vi "_RT Global.vi"() -> ()   [LabVIEW 2018]
uses:
  Type/_RT Instrument 2.ctl
  Type/_RT Configuration 2.ctl
  Type/_RT Startup Options.ctl
  Type/_RT Instrument State.ctl
  Type/FPGA Typedef.ctl
panel:
  out "Leybold Pump ON":bool
  out "Tuning Error Generated":bool
  out "Exhaust gas error":bool
  out "ScanParam":bool
  out "UseLeybold":bool
  out "FPGA Ref":T1
  out "IgnoreError":bool
  out "Simulation":bool
  out "Single Source":bool
  out "FPGA semaphore":T2
  out "Ele On":bool
  out "semaphore":T2
  out "RT Time(s)":dbl=432.2503070831299
  out "ADC Values":i32[](array[numeric])=[0, 0, 0, 0, 0, 0, 0, 0, 0, 0, 0, 0, 0, 0, 0, 0, 0, 0, 0, 0, 0, 0, 0, 0, 0, 0, 0, 0, 0, 0, 0, 0, 0, 0, 0, 0, 0, 0, 0, 0, 0, 0, 0, 0, 0, 0, 0, 0, 0, 0, 0, 0, 0, 0, 0, 0, 0, 0, 0, 0, 0, 0, 0, 0, 0, 0, 0, 0, 0, 0, 0, 0, 0, 0, 0, 0, 0, 0, 0, 0, 0, 0, 0, 0, 0, 0, 0, 0, 0, 0, 0, 0, 0, 0, 0, 0, 0, 0, 0, 0, 0, 0, 0, 0, 0, 0, 0, 0, 0, 0, 0, 0, 0, 0, 0, 0, 0, 0, 0, 0, 0, 0, 1, 0, 1, 0, 0, 0]
  out "StartupMode":u8=2
  out "InstrState":T3=enum."Mass Spectrometer is Off"
  in  "ADC Table":T4[](array[typedef])=[{"Name"="DET HORN, 6KV", "Ch#"=0, "Min"=0.0, "Max"=0.0, "Def+"=0.0, "Def-"=0.0, "Offset"=0.0, "Slope"=33.0, "Type"=0, "Description"="", "SettleT"=0.0}, {"Name"="DET BIAS, KV", "Ch#"=0, "Min"=0.0, "Max"=0.0, "Def+"=0.0, "Def-"=0.0, "Offset"=0.0, "Slope"=33.0, "Type"=0, "Description"="", "SettleT"=0.0}, {"Name"="Discriminator", "Ch#"=0, "Min"=0.0, "Max"=0.0, "Def+"=0.0, "Def-"=0.0, "Offset"=4.0, "Slope"=1100.0, "Type"=0, "Description"="", "SettleT"=0.0}, {"Name"="DET Spare4", "Ch#"=0, "Min"=0.0, "Max"=0.0, "Def+"=0.0, "Def-"=0.0, "Offset"=0.0, "Slope"=1.0, "Type"=0, "Description"="", "SettleT"=0.0}, {"Name"="DET Spare5", "Ch#"=0, "Min"=0.0, "Max"=0.0, "Def+"=0.0, "Def-"=0.0, "Offset"=0.0, "Slope"=1.0, "Type"=0, "Description"="", "SettleT"=0.0}, {"Name"="DET Spare6", "Ch#"=0, "Min"=0.0, "Max"=0.0, "Def+"=0.0, "Def-"=0.0, "Offset"=0.0, "Slope"=1.0, "Type"=0, "Description"="", "SettleT"=0.0}, {"Name"="DET Spare7", "Ch#"=0, "Min"=0.0, "Max"=0.0, "Def+"=0.0, "Def-"=0.0, "Offset"=0.0, "Slope"=1.0, "Type"=0, "Description"="", "SettleT"=0.0}, {"Name"="DET Spare8", "Ch#"=0, "Min"=0.0, "Max"=0.0, "Def+"=0.0, "Def-"=0.0, "Offset"=0.0, "Slope"=1.0, "Type"=0, "Description"="", "SettleT"=0.0}, {"Name"="LV PS CUR, 10A", "Ch#"=0, "Min"=0.0, "Max"=0.0, "Def+"=0.0, "Def-"=0.0, "Offset"=0.0, "Slope"=1.0, "Type"=0, "Description"="", "SettleT"=0.0}, {"Name"="RPUMP CUR, 30A", "Ch#"=0, "Min"=0.0, "Max"=0.0, "Def+"=0.0, "Def-"=0.0, "Offset"=0.0, "Slope"=1.0, "Type"=0, "Description"="", "SettleT"=0.0}, {"Name"="AC box Spare3", "Ch#"=0, "Min"=0.0, "Max"=0.0, "Def+"=0.0, "Def-"=0.0, "Offset"=0.0, "Slope"=1.0, "Type"=0, "Description"="", "SettleT"=0.0}, {"Name"="AC box Spare4", "Ch#"=0, "Min"=0.0, "Max"=0.0, "Def+"=0.0, "Def-"=0.0, "Offset"=0.0, "Slope"=1.0, "Type"=0, "Description"="", "SettleT"=0.0}, {"Name"="AC box Spare5", "Ch#"=0, "Min"=0.0, "Max"=0.0, "Def+"=0.0, "Def-"=0.0, "Offset"=0.0, "Slope"=1.0, "Type"=0, "Description"="", "SettleT"=0.0}, {"Name"="AC box Spare6", "Ch#"=0, "Min"=0.0, "Max"=0.0, "Def+"=0.0, "Def-"=0.0, "Offset"=0.0, "Slope"=1.0, "Type"=0, "Description"="", "SettleT"=0.0}, {"Name"="HTR PS CUR, 10A", "Ch#"=0, "Min"=0.0, "Max"=0.0, "Def+"=0.0, "Def-"=0.0, "Offset"=0.0, "Slope"=1.0, "Type"=0, "Description"="", "SettleT"=0.0}, {"Name"="TRB PS CUR, 5A", "Ch#"=0, "Min"=0.0, "Max"=0.0, "Def+"=0.0, "Def-"=0.0, "Offset"=0.0, "Slope"=1.0, "Type"=0, "Description"="", "SettleT"=0.0}, {"Name"="Q1 DC POLE A, V", "Ch#"=0, "Min"=0.0, "Max"=0.0, "Def+"=0.0, "Def-"=0.0, "Offset"=0.5, "Slope"=402.0, "Type"=0, "Description"="", "SettleT"=0.0}, {"Name"="Q1 DC POLE B, V", "Ch#"=0, "Min"=0.0, "Max"=0.0, "Def+"=0.0, "Def-"=0.0, "Offset"=0.5, "Slope"=402.0, "Type"=0, "Description"="", "SettleT"=0.0}, {"Name"="Q2 DC POLE A, V", "Ch#"=0, "Min"=0.0, "Max"=0.0, "Def+"=0.0, "Def-"=0.0, "Offset"=0.5, "Slope"=402.0, "Type"=0, "Description"="", "SettleT"=0.0}, {"Name"="Q2 DC POLE B, V", "Ch#"=0, "Min"=0.0, "Max"=0.0, "Def+"=0.0, "Def-"=0.0, "Offset"=0.5, "Slope"=402.0, "Type"=0, "Description"="", "SettleT"=0.0}, {"Name"="DC Spare5", "Ch#"=0, "Min"=0.0, "Max"=0.0, "Def+"=0.0, "Def-"=0.0, "Offset"=0.0, "Slope"=1.0, "Type"=0, "Description"="", "SettleT"=0.0}, {"Name"="DC Spare6", "Ch#"=0, "Min"=0.0, "Max"=0.0, "Def+"=0.0, "Def-"=0.0, "Offset"=0.0, "Slope"=1.0, "Type"=0, "Description"="", "SettleT"=0.0}, {"Name"="DC Spare7", "Ch#"=0, "Min"=0.0, "Max"=0.0, "Def+"=0.0, "Def-"=0.0, "Offset"=0.0, "Slope"=1.0, "Type"=0, "Description"="", "SettleT"=0.0}, {"Name"="DC Spare8", "Ch#"=0, "Min"=0.0, "Max"=0.0, "Def+"=0.0, "Def-"=0.0, "Offset"=0.0, "Slope"=1.0, "Type"=0, "Description"="", "SettleT"=0.0}, {"Name"="Q2 RF Pk-Pk, V", "Ch#"=0, "Min"=0.0, "Max"=0.0, "Def+"=0.0, "Def-"=0.0, "Offset"=0.0, "Slope"=-1208.0, "Type"=0, "Description"="", "SettleT"=0.0}, {"Name"="Q2 RF HS1 TEMP, C", "Ch#"=0, "Min"=0.0, "Max"=90.0, "Def+"=0.0, "Def-"=0.0, "Offset"=0.0, "Slope"=100.0, "Type"=0, "Description"="", "SettleT"=0.0}, {"Name"="Q2 RF HS2 TEMP, C", "Ch#"=0, "Min"=0.0, "Max"=0.0, "Def+"=0.0, "Def-"=0.0, "Offset"=0.0, "Slope"=100.0, "Type"=0, "Description"="", "SettleT"=0.0}, {"Name"="Q2 TUNING DC, V", "Ch#"=0, "Min"=0.0, "Max"=0.0, "Def+"=0.0, "Def-"=0.0, "Offset"=0.0, "Slope"=3.0, "Type"=0, "Description"="", "SettleT"=0.0}, {"Name"="Q2 RF Spare5", "Ch#"=0, "Min"=0.0, "Max"=0.0, "Def+"=0.0, "Def-"=0.0, "Offset"=0.0, "Slope"=1.0, "Type"=0, "Description"="", "SettleT"=0.0}, {"Name"="Q2 RF Spare6", "Ch#"=0, "Min"=0.0, "Max"=0.0, "Def+"=0.0, "Def-"=0.0, "Offset"=0.0, "Slope"=1.0, "Type"=0, "Description"="", "SettleT"=0.0}, {"Name"="Q2 RF Spare7", "Ch#"=0, "Min"=0.0, "Max"=0.0, "Def+"=0.0, "Def-"=0.0, "Offset"=0.0, "Slope"=1.0, "Type"=0, "Description"="", "SettleT"=0.0}, {"Name"="Q2 RF Spare8", "Ch#"=0, "Min"=0.0, "Max"=0.0, "Def+"=0.0, "Def-"=0.0, "Offset"=0.0, "Slope"=1.0, "Type"=0, "Description"="", "SettleT"=0.0}, {"Name"="CC AF +/-400, V", "Ch#"=0, "Min"=0.0, "Max"=0.0, "Def+"=0.0, "Def-"=0.0, "Offset"=1.0, "Slope"=402.0, "Type"=0, "Description"="", "SettleT"=0.0}, {"Name"="L2 +/-400, V", "Ch#"=0, "Min"=0.0, "Max"=0.0, "Def+"=0.0, "Def-"=0.0, "Offset"=1.0, "Slope"=402.0, "Type"=0, "Description"="", "SettleT"=0.0}, {"Name"="PF +/-400, V", "Ch#"=0, "Min"=0.0, "Max"=0.0, "Def+"=0.0, "Def-"=0.0, "Offset"=1.0, "Slope"=402.0, "Type"=0, "Description"="", "SettleT"=0.0}, {"Name"="CC L1 +/-400, V", "Ch#"=0, "Min"=0.0, "Max"=0.0, "Def+"=0.0, "Def-"=0.0, "Offset"=1.0, "Slope"=402.0, "Type"=0, "Description"="", "SettleT"=0.0}, {"Name"="CC L2 +/-400, V", "Ch#"=0, "Min"=0.0, "Max"=0.0, "Def+"=0.0, "Def-"=0.0, "Offset"=1.0, "Slope"=402.0, "Type"=0, "Description"="", "SettleT"=0.0}, {"Name"="CC L3 +/-400, V", "Ch#"=0, "Min"=0.0, "Max"=0.0, "Def+"=0.0, "Def-"=0.0, "Offset"=1.0, "Slope"=404.0, "Type"=0, "Description"="", "SettleT"=0.0}, {"Name"="CC L4 +/-400, V", "Ch#"=0, "Min"=0.0, "Max"=0.0, "Def+"=0.0, "Def-"=0.0, "Offset"=1.0, "Slope"=404.0, "Type"=0, "Description"="", "SettleT"=0.0}, {"Name"="ID +/-400, V", "Ch#"=0, "Min"=0.0, "Max"=0.0, "Def+"=0.0, "Def-"=0.0, "Offset"=1.0, "Slope"=404.0, "Type"=0, "Description"="", "SettleT"=0.0}, {"Name"="L1 +/-400, V", "Ch#"=0, "Min"=0.0, "Max"=0.0, "Def+"=0.0, "Def-"=0.0, "Offset"=1.0, "Slope"=400.0, "Type"=0, "Description"="", "SettleT"=0.0}, {"Name"="M1 +/-400, V", "Ch#"=0, "Min"=0.0, "Max"=0.0, "Def+"=0.0, "Def-"=0.0, "Offset"=1.0, "Slope"=402.0, "Type"=0, "Description"="", "SettleT"=0.0}, {"Name"="EV +/-400, V", "Ch#"=0, "Min"=0.0, "Max"=0.0, "Def+"=0.0, "Def-"=0.0, "Offset"=4.0, "Slope"=404.0, "Type"=0, "Description"="", "SettleT"=0.0}, {"Name"="Spare +/-400, V", "Ch#"=0, "Min"=0.0, "Max"=0.0, "Def+"=0.0, "Def-"=0.0, "Offset"=1.0, "Slope"=402.0, "Type"=0, "Description"="", "SettleT"=0.0}, {"Name"="M2 +/-400, V", "Ch#"=0, "Min"=0.0, "Max"=0.0, "Def+"=0.0, "Def-"=0.0, "Offset"=3.0, "Slope"=404.0, "Type"=0, "Description"="", "SettleT"=0.0}, {"Name"="CC +/-400, V", "Ch#"=0, "Min"=0.0, "Max"=0.0, "Def+"=0.0, "Def-"=0.0, "Offset"=1.0, "Slope"=404.0, "Type"=0, "Description"="", "SettleT"=0.0}, {"Name"="Spare +/-400, V", "Ch#"=0, "Min"=0.0, "Max"=0.0, "Def+"=0.0, "Def-"=0.0, "Offset"=0.0, "Slope"=404.0, "Type"=0, "Description"="", "SettleT"=0.0}, {"Name"="Spare +/-400, V", "Ch#"=0, "Min"=0.0, "Max"=0.0, "Def+"=0.0, "Def-"=0.0, "Offset"=-1.5, "Slope"=404.0, "Type"=0, "Description"="", "SettleT"=0.0}, {"Name"="Q1 RF Pk-Pk, V", "Ch#"=0, "Min"=0.0, "Max"=0.0, "Def+"=0.0, "Def-"=0.0, "Offset"=0.0, "Slope"=-1221.0, "Type"=0, "Description"="", "SettleT"=0.0}, {"Name"="Q1 RF HS1 TEMP, C", "Ch#"=0, "Min"=0.0, "Max"=0.0, "Def+"=0.0, "Def-"=0.0, "Offset"=0.0, "Slope"=100.0, "Type"=0, "Description"="", "SettleT"=0.0}, {"Name"="Q1 RF HS2 TEMP, C", "Ch#"=0, "Min"=0.0, "Max"=0.0, "Def+"=0.0, "Def-"=0.0, "Offset"=0.0, "Slope"=100.0, "Type"=0, "Description"="", "SettleT"=0.0}, {"Name"="Q1 TUNING DC, V", "Ch#"=0, "Min"=0.0, "Max"=0.0, "Def+"=0.0, "Def-"=0.0, "Offset"=0.0, "Slope"=3.0, "Type"=0, "Description"="", "SettleT"=0.0}, {"Name"="Q1 RF Spare5", "Ch#"=0, "Min"=0.0, "Max"=0.0, "Def+"=0.0, "Def-"=0.0, "Offset"=0.0, "Slope"=1.0, "Type"=0, "Description"="", "SettleT"=0.0}, {"Name"="Q1 RF Spare6", "Ch#"=0, "Min"=0.0, "Max"=0.0, "Def+"=0.0, "Def-"=0.0, "Offset"=0.0, "Slope"=1.0, "Type"=0, "Description"="", "SettleT"=0.0}, {"Name"="Q1 RF Spare7", "Ch#"=0, "Min"=0.0, "Max"=0.0, "Def+"=0.0, "Def-"=0.0, "Offset"=0.0, "Slope"=1.0, "Type"=0, "Description"="", "SettleT"=0.0}, {"Name"="Q1 RF Spare8", "Ch#"=0, "Min"=0.0, "Max"=0.0, "Def+"=0.0, "Def-"=0.0, "Offset"=0.0, "Slope"=1.0, "Type"=0, "Description"="", "SettleT"=0.0}, {"Name"="M1 RF Pk-Pk, V", "Ch#"=0, "Min"=0.0, "Max"=0.0, "Def+"=0.0, "Def-"=0.0, "Offset"=0.0, "Slope"=-885.0, "Type"=0, "Description"="", "SettleT"=0.0}, {"Name"="M1 RF HS1 TEMP, C", "Ch#"=0, "Min"=0.0, "Max"=0.0, "Def+"=0.0, "Def-"=0.0, "Offset"=0.0, "Slope"=100.0, "Type"=0, "Description"="", "SettleT"=0.0}, {"Name"="M1 RF HS2 TEMP, C", "Ch#"=0, "Min"=0.0, "Max"=0.0, "Def+"=0.0, "Def-"=0.0, "Offset"=0.0, "Slope"=100.0, "Type"=0, "Description"="", "SettleT"=0.0}, {"Name"="M1 TUNING DC, V", "Ch#"=0, "Min"=0.0, "Max"=0.0, "Def+"=0.0, "Def-"=0.0, "Offset"=0.0, "Slope"=3.0, "Type"=0, "Description"="", "SettleT"=0.0}, {"Name"="M1 RF Spare5", "Ch#"=0, "Min"=0.0, "Max"=0.0, "Def+"=0.0, "Def-"=0.0, "Offset"=0.0, "Slope"=1.0, "Type"=0, "Description"="", "SettleT"=0.0}, {"Name"="M1 RF Spare6", "Ch#"=0, "Min"=0.0, "Max"=0.0, "Def+"=0.0, "Def-"=0.0, "Offset"=0.0, "Slope"=1.0, "Type"=0, "Description"="", "SettleT"=0.0}, {"Name"="M1 RF Spare7", "Ch#"=0, "Min"=0.0, "Max"=0.0, "Def+"=0.0, "Def-"=0.0, "Offset"=0.0, "Slope"=1.0, "Type"=0, "Description"="", "SettleT"=0.0}, {"Name"="M1 RF Spare8", "Ch#"=0, "Min"=0.0, "Max"=0.0, "Def+"=0.0, "Def-"=0.0, "Offset"=0.0, "Slope"=1.0, "Type"=0, "Description"="", "SettleT"=0.0}, {"Name"="Drying Gas Output, V", "Ch#"=0, "Min"=0.0, "Max"=0.0, "Def+"=0.0, "Def-"=0.0, "Offset"=0.0, "Slope"=1.0, "Type"=0, "Description"="", "SettleT"=0.0}, {"Name"="Neb Gas 1 Out, V", "Ch#"=0, "Min"=0.0, "Max"=0.0, "Def+"=0.0, "Def-"=0.0, "Offset"=0.0, "Slope"=1.0, "Type"=0, "Description"="", "SettleT"=0.0}, {"Name"="Neb Gas 2 Out, V", "Ch#"=0, "Min"=0.0, "Max"=0.0, "Def+"=0.0, "Def-"=0.0, "Offset"=0.0, "Slope"=1.0, "Type"=0, "Description"="", "SettleT"=0.0}, {"Name"="Heater Gas 1 Out, V", "Ch#"=0, "Min"=0.0, "Max"=0.0, "Def+"=0.0, "Def-"=0.0, "Offset"=0.0, "Slope"=1.0, "Type"=0, "Description"="", "SettleT"=0.0}, {"Name"="Heater Gas 2 Out, V", "Ch#"=0, "Min"=0.0, "Max"=0.0, "Def+"=0.0, "Def-"=0.0, "Offset"=0.0, "Slope"=1.0, "Type"=0, "Description"="", "SettleT"=0.0}, {"Name"="Gas box Spare6", "Ch#"=0, "Min"=0.0, "Max"=0.0, "Def+"=0.0, "Def-"=0.0, "Offset"=0.0, "Slope"=1.0, "Type"=0, "Description"="", "SettleT"=0.0}, {"Name"="SourceExhaust on/off", "Ch#"=0, "Min"=0.0, "Max"=0.0, "Def+"=0.0, "Def-"=0.0, "Offset"=0.0, "Slope"=1.0, "Type"=0, "Description"="", "SettleT"=0.0}, {"Name"="CC Gas 0-18 V, V", "Ch#"=0, "Min"=0.0, "Max"=0.0, "Def+"=0.0, "Def-"=0.0, "Offset"=0.0, "Slope"=1.0, "Type"=0, "Description"="", "SettleT"=0.0}, {"Name"="S Exhaust reading", "Ch#"=0, "Min"=0.0, "Max"=0.0, "Def+"=0.0, "Def-"=0.0, "Offset"=0.0, "Slope"=1.0, "Type"=0, "Description"="", "SettleT"=0.0}, {"Name"="Press Spare2", "Ch#"=0, "Min"=0.0, "Max"=0.0, "Def+"=0.0, "Def-"=0.0, "Offset"=0.0, "Slope"=1.0, "Type"=0, "Description"="", "SettleT"=0.0}, {"Name"="Foreline Press, torr", "Ch#"=0, "Min"=0.0, "Max"=0.0, "Def+"=0.0, "Def-"=0.0, "Offset"=0.0, "Slope"=45.0, "Type"=0, "Description"="", "SettleT"=0.0}, {"Name"="Press Spare4", "Ch#"=0, "Min"=0.0, "Max"=0.0, "Def+"=0.0, "Def-"=0.0, "Offset"=0.0, "Slope"=1.0, "Type"=0, "Description"="", "SettleT"=0.0}, {"Name"="Drying Gas Input P (V)", "Ch#"=0, "Min"=0.0, "Max"=0.0, "Def+"=0.0, "Def-"=0.0, "Offset"=-12.5, "Slope"=25.0, "Type"=0, "Description"="", "SettleT"=0.0}, {"Name"="Press Spare6", "Ch#"=0, "Min"=0.0, "Max"=0.0, "Def+"=0.0, "Def-"=0.0, "Offset"=0.0, "Slope"=1.0, "Type"=0, "Description"="", "SettleT"=0.0}, {"Name"="Gas Manifold Input P (V)", "Ch#"=0, "Min"=0.0, "Max"=0.0, "Def+"=0.0, "Def-"=0.0, "Offset"=-12.5, "Slope"=25.0, "Type"=0, "Description"="", "SettleT"=0.0}, {"Name"="Press Spare8", "Ch#"=0, "Min"=0.0, "Max"=0.0, "Def+"=0.0, "Def-"=0.0, "Offset"=0.0, "Slope"=1.0, "Type"=0, "Description"="", "SettleT"=0.0}, {"Name"="24V (+)", "Ch#"=0, "Min"=0.0, "Max"=0.0, "Def+"=0.0, "Def-"=0.0, "Offset"=0.0, "Slope"=5.0, "Type"=0, "Description"="", "SettleT"=0.0}, {"Name"="28V (+)", "Ch#"=0, "Min"=0.0, "Max"=0.0, "Def+"=0.0, "Def-"=0.0, "Offset"=0.0, "Slope"=5.6, "Type"=0, "Description"="", "SettleT"=0.0}, {"Name"="28V (-)", "Ch#"=0, "Min"=0.0, "Max"=0.0, "Def+"=0.0, "Def-"=0.0, "Offset"=0.0, "Slope"=5.6, "Type"=0, "Description"="", "SettleT"=0.0}, {"Name"="60V (+)", "Ch#"=0, "Min"=0.0, "Max"=0.0, "Def+"=0.0, "Def-"=0.0, "Offset"=0.0, "Slope"=12.0, "Type"=0, "Description"="", "SettleT"=0.0}, {"Name"="48V (+)", "Ch#"=0, "Min"=0.0, "Max"=0.0, "Def+"=0.0, "Def-"=0.0, "Offset"=0.0, "Slope"=9.6, "Type"=0, "Description"="", "SettleT"=0.0}, {"Name"="24V (-)", "Ch#"=0, "Min"=0.0, "Max"=0.0, "Def+"=0.0, "Def-"=0.0, "Offset"=0.0, "Slope"=5.0, "Type"=0, "Description"="", "SettleT"=0.0}, {"Name"="15V (+)", "Ch#"=0, "Min"=0.0, "Max"=0.0, "Def+"=0.0, "Def-"=0.0, "Offset"=0.0, "Slope"=3.0, "Type"=0, "Description"="", "SettleT"=0.0}, {"Name"="15V (-)", "Ch#"=0, "Min"=0.0, "Max"=0.0, "Def+"=0.0, "Def-"=0.0, "Offset"=0.0, "Slope"=3.0, "Type"=0, "Description"="", "SettleT"=0.0}, {"Name"="Lens Board 2 Pos (V)", "Ch#"=0, "Min"=0.0, "Max"=0.0, "Def+"=0.0, "Def-"=0.0, "Offset"=0.0, "Slope"=100.0, "Type"=0, "Description"="", "SettleT"=0.0}, {"Name"="Lens Board 2 Neg (V)", "Ch#"=0, "Min"=0.0, "Max"=0.0, "Def+"=0.0, "Def-"=0.0, "Offset"=0.0, "Slope"=100.0, "Type"=0, "Description"="", "SettleT"=0.0}, {"Name"="Lens Board 2 Pos (A)", "Ch#"=0, "Min"=0.0, "Max"=0.0, "Def+"=0.0, "Def-"=0.0, "Offset"=0.0, "Slope"=1.0, "Type"=0, "Description"="", "SettleT"=0.0}, {"Name"="Lens Board 2 Neg (A)", "Ch#"=0, "Min"=0.0, "Max"=0.0, "Def+"=0.0, "Def-"=0.0, "Offset"=0.0, "Slope"=1.0, "Type"=0, "Description"="", "SettleT"=0.0}, {"Name"="L1-ADC12-5", "Ch#"=0, "Min"=0.0, "Max"=0.0, "Def+"=0.0, "Def-"=0.0, "Offset"=0.0, "Slope"=1.0, "Type"=0, "Description"="", "SettleT"=0.0}, {"Name"="L1-ADC12-6", "Ch#"=0, "Min"=0.0, "Max"=0.0, "Def+"=0.0, "Def-"=0.0, "Offset"=0.0, "Slope"=1.0, "Type"=0, "Description"="", "SettleT"=0.0}, {"Name"="L1-ADC12-7", "Ch#"=0, "Min"=0.0, "Max"=0.0, "Def+"=0.0, "Def-"=0.0, "Offset"=0.0, "Slope"=1.0, "Type"=0, "Description"="", "SettleT"=0.0}, {"Name"="L1-ADC12-8", "Ch#"=0, "Min"=0.0, "Max"=0.0, "Def+"=0.0, "Def-"=0.0, "Offset"=0.0, "Slope"=1.0, "Type"=0, "Description"="", "SettleT"=0.0}, {"Name"="Lens Board 1 Pos (V)", "Ch#"=0, "Min"=0.0, "Max"=0.0, "Def+"=0.0, "Def-"=0.0, "Offset"=0.0, "Slope"=100.0, "Type"=0, "Description"="", "SettleT"=0.0}, {"Name"="Lens Board 1 Neg (V)", "Ch#"=0, "Min"=0.0, "Max"=0.0, "Def+"=0.0, "Def-"=0.0, "Offset"=0.0, "Slope"=100.0, "Type"=0, "Description"="", "SettleT"=0.0}, {"Name"="Lens Board 1 Pos (A)", "Ch#"=0, "Min"=0.0, "Max"=0.0, "Def+"=0.0, "Def-"=0.0, "Offset"=0.0, "Slope"=1.0, "Type"=0, "Description"="", "SettleT"=0.0}, {"Name"="Lens Board 2 Neg (A)", "Ch#"=0, "Min"=0.0, "Max"=0.0, "Def+"=0.0, "Def-"=0.0, "Offset"=0.0, "Slope"=1.0, "Type"=0, "Description"="", "SettleT"=0.0}, {"Name"="L3-ADC13-5", "Ch#"=0, "Min"=0.0, "Max"=0.0, "Def+"=0.0, "Def-"=0.0, "Offset"=0.0, "Slope"=1.0, "Type"=0, "Description"="", "SettleT"=0.0}, {"Name"="L3-ADC13-6", "Ch#"=0, "Min"=0.0, "Max"=0.0, "Def+"=0.0, "Def-"=0.0, "Offset"=0.0, "Slope"=1.0, "Type"=0, "Description"="", "SettleT"=0.0}, {"Name"="L3-ADC13-7", "Ch#"=0, "Min"=0.0, "Max"=0.0, "Def+"=0.0, "Def-"=0.0, "Offset"=0.0, "Slope"=1.0, "Type"=0, "Description"="", "SettleT"=0.0}, {"Name"="L3-ADC13-8", "Ch#"=0, "Min"=0.0, "Max"=0.0, "Def+"=0.0, "Def-"=0.0, "Offset"=0.0, "Slope"=1.0, "Type"=0, "Description"="", "SettleT"=0.0}, {"Name"="CAP POS", "Ch#"=0, "Min"=0.0, "Max"=0.0, "Def+"=0.0, "Def-"=0.0, "Offset"=0.0, "Slope"=13.9, "Type"=0, "Description"="", "SettleT"=0.0}, {"Name"="HSID T", "Ch#"=0, "Min"=0.0, "Max"=0.0, "Def+"=0.0, "Def-"=0.0, "Offset"=0.0, "Slope"=1.0, "Type"=0, "Description"="", "SettleT"=0.0}, {"Name"="CD Corona POS", "Ch#"=0, "Min"=0.0, "Max"=0.0, "Def+"=0.0, "Def-"=0.0, "Offset"=0.0, "Slope"=1.0, "Type"=0, "Description"="", "SettleT"=0.0}, {"Name"="ISV1 POS", "Ch#"=0, "Min"=0.0, "Max"=0.0, "Def+"=0.0, "Def-"=0.0, "Offset"=0.0, "Slope"=42.599998, "Type"=0, "Description"="", "SettleT"=0.0}, {"Name"="Probe2 Temp", "Ch#"=0, "Min"=0.0, "Max"=0.0, "Def+"=0.0, "Def-"=0.0, "Offset"=0.0, "Slope"=1.0, "Type"=0, "Description"="", "SettleT"=0.0}, {"Name"="ISV2 POS", "Ch#"=0, "Min"=0.0, "Max"=0.0, "Def+"=0.0, "Def-"=0.0, "Offset"=0.0, "Slope"=42.639999, "Type"=0, "Description"="", "SettleT"=0.0}, {"Name"="Probe1 Temp", "Ch#"=0, "Min"=0.0, "Max"=0.0, "Def+"=0.0, "Def-"=0.0, "Offset"=0.0, "Slope"=1.0, "Type"=0, "Description"="", "SettleT"=0.0}, {"Name"="PIC 87", "Ch#"=0, "Min"=0.0, "Max"=0.0, "Def+"=0.0, "Def-"=0.0, "Offset"=0.0, "Slope"=1.0, "Type"=0, "Description"="", "SettleT"=0.0}, {"Name"="PIC 88", "Ch#"=0, "Min"=0.0, "Max"=0.0, "Def+"=0.0, "Def-"=0.0, "Offset"=0.0, "Slope"=1.0, "Type"=0, "Description"="", "SettleT"=0.0}, {"Name"="PROBE 1 ID", "Ch#"=0, "Min"=0.0, "Max"=0.0, "Def+"=0.0, "Def-"=0.0, "Offset"=0.0, "Slope"=1.0, "Type"=0, "Description"="", "SettleT"=0.0}, {"Name"="PROBE 2 ID", "Ch#"=0, "Min"=0.0, "Max"=0.0, "Def+"=0.0, "Def-"=0.0, "Offset"=0.0, "Slope"=1.0, "Type"=0, "Description"="", "SettleT"=0.0}, {"Name"="ISV1 NEG", "Ch#"=0, "Min"=0.0, "Max"=0.0, "Def+"=0.0, "Def-"=0.0, "Offset"=0.0, "Slope"=-42.639999, "Type"=0, "Description"="", "SettleT"=0.0}, {"Name"="ISV2 NEG", "Ch#"=0, "Min"=0.0, "Max"=0.0, "Def+"=0.0, "Def-"=0.0, "Offset"=0.0, "Slope"=-42.639999, "Type"=0, "Description"="", "SettleT"=0.0}, {"Name"="CAP NEG", "Ch#"=0, "Min"=0.0, "Max"=0.0, "Def+"=0.0, "Def-"=0.0, "Offset"=0.0, "Slope"=-13.9, "Type"=0, "Description"="", "SettleT"=0.0}, {"Name"="CD Corona NEG", "Ch#"=0, "Min"=0.0, "Max"=0.0, "Def+"=0.0, "Def-"=0.0, "Offset"=0.0, "Slope"=1.0, "Type"=0, "Description"="", "SettleT"=0.0}, {"Name"="VAC Gauge", "Ch#"=0, "Min"=0.0, "Max"=0.0, "Def+"=0.0, "Def-"=0.0, "Offset"=0.0, "Slope"=1.0, "Type"=0, "Description"="", "SettleT"=0.0}, {"Name"="Door Interlock", "Ch#"=0, "Min"=0.0, "Max"=0.0, "Def+"=0.0, "Def-"=0.0, "Offset"=0.0, "Slope"=1.0, "Type"=0, "Description"="", "SettleT"=0.0}, {"Name"="Vacuum Ready", "Ch#"=0, "Min"=0.0, "Max"=0.0, "Def+"=0.0, "Def-"=0.0, "Offset"=0.0, "Slope"=1.0, "Type"=0, "Description"="", "SettleT"=0.0}, {"Name"="LC1 Out1 Hold", "Ch#"=0, "Min"=0.0, "Max"=0.0, "Def+"=0.0, "Def-"=0.0, "Offset"=0.0, "Slope"=1.0, "Type"=0, "Description"="", "SettleT"=0.0}, {"Name"="LC1 Out2 Stop", "Ch#"=0, "Min"=0.0, "Max"=0.0, "Def+"=0.0, "Def-"=0.0, "Offset"=0.0, "Slope"=1.0, "Type"=0, "Description"="", "SettleT"=0.0}, {"Name"="LC2 Out1 Hold", "Ch#"=0, "Min"=0.0, "Max"=0.0, "Def+"=0.0, "Def-"=0.0, "Offset"=0.0, "Slope"=1.0, "Type"=0, "Description"="", "SettleT"=0.0}, {"Name"="LC2 Out2 Stop", "Ch#"=0, "Min"=0.0, "Max"=0.0, "Def+"=0.0, "Def-"=0.0, "Offset"=0.0, "Slope"=1.0, "Type"=0, "Description"="", "SettleT"=0.0}, {"Name"="LC1 In", "Ch#"=0, "Min"=0.0, "Max"=0.0, "Def+"=0.0, "Def-"=0.0, "Offset"=0.0, "Slope"=1.0, "Type"=0, "Description"="", "SettleT"=0.0}, {"Name"="LC2 In", "Ch#"=0, "Min"=0.0, "Max"=0.0, "Def+"=0.0, "Def-"=0.0, "Offset"=0.0, "Slope"=1.0, "Type"=0, "Description"="", "SettleT"=0.0}] {"Slope" format="%#.2f"}
  out "StartupOptions":T5={"Door"=TRUE, "Curtain"=TRUE, "Pressure"=TRUE, "Turbo"=TRUE, "SysPoll"=TRUE, "GasFlag"=TRUE, "SourceExhaust"=TRUE}
  out "ErrorMsg":string
  out "Q2 -Res Lo":dbl[][](array[numeric])=[[0.0, 32500.0], [45.0, 33050.0], [514.1, 36000.77464788732], [585.4, 36552.29226361032], [933.6, 38547.70773638968], [1223.8, 40148.896492931395], [1456.0, 41430.06819957849], [1500.0, 41672.83975467096]] format="%.2f"
  out "Q2 -Res Med":dbl[][](array[numeric])=[[0.0, 32500.0], [45.0, 33050.0], [514.1, 36000.77464788732], [585.4, 36552.29226361032], [933.6, 38547.70773638968], [1223.8, 40148.896492931395], [1456.0, 41430.06819957849], [1500.0, 41672.83975467096]] format="%.2f"
  out "Q1 -Res Lo":dbl[][](array[numeric])=[[0.0, 33265.24137931035], [45.0, 33749.379310344826], [514.1, 37400.0], [585.4, 37795.114503816796], [933.6, 39960.51724137931], [1223.8, 41711.724137931036], [1456.0, 43201.15291898124], [1500.0, 43600.0]] format="%.2f"
  out "Q1 -Res Med":dbl[][](array[numeric])=[[0.0, 33265.24137931035], [45.0, 33749.379310344826], [514.1, 37400.0], [585.4, 37795.114503816796], [933.6, 39960.51724137931], [1223.8, 41711.724137931036], [1456.0, 43201.15291898124], [1500.0, 43600.0]] format="%.2f"
  out "Q2 -Res Hi":dbl[][](array[numeric])=[[0.0, 32500.0], [45.0, 33050.0], [514.1, 36000.77464788732], [585.4, 36552.29226361032], [933.6, 38547.70773638968], [1223.8, 40148.896492931395], [1456.0, 41430.06819957849], [1500.0, 41672.83975467096]] format="%.2f"
  out "Q1 -Res Hi":dbl[][](array[numeric])=[[0.0, 33265.24137931035], [45.0, 33749.379310344826], [514.1, 37400.0], [585.4, 37795.114503816796], [933.6, 39960.51724137931], [1223.8, 41711.724137931036], [1456.0, 43201.15291898124], [1500.0, 43600.0]] format="%.2f"
  out "Q2 POL":bool
  out "Q1 POL":bool
  out "Q2 -Cal":dbl[][](array[numeric])=[[0.0, 0.0], [45.0, 6064.168025288581], [514.1, 71104.0], [585.4, 80965.0], [933.6, 129151.03618609994], [1223.8, 169370.96671193905], [1456.0, 201691.0], [1500.0, 207815.38184614418]] format="%.2f"
  out "Q1 -Cal":dbl[][](array[numeric])=[[0.0, 0.0], [45.0, 6058.0], [514.1, 70943.72007379876], [585.4, 80765.52138069598], [933.6, 128993.0], [1223.8, 169105.4900068918], [1456.0, 201276.0], [1500.0, 207372.04840524014]] format="%.2f"
  in  "Configuration 2":T6={"Table"=[{"Name"="Q1 RF", "Ch#"=1, "Min"=0.0, "Max"=1500.0, "Def+"=400.0, "Def-"=400.0, "Offset"=0.0, "Slope"=218.45, "Type"=64, "Description"="Quadrupole 1 RF", "SettleT"=5.0}, {"Name"="Q1 DC", "Ch#"=4, "Min"=0.0, "Max"=1500.0, "Def+"=600.0, "Def-"=600.0, "Offset"=0.0, "Slope"=218.45, "Type"=64, "Description"="Quadrupole 1 DC", "SettleT"=5.0}, {"Name"="Q1 RR", "Ch#"=7, "Min"=0.0, "Max"=64000.0, "Def+"=32000.0, "Def-"=32000.0, "Offset"=32768.0, "Slope"=-1.0, "Type"=64, "Description"="Quadrupole 1 PW", "SettleT"=5.0}, {"Name"="Q2 RF", "Ch#"=2, "Min"=0.0, "Max"=1500.0, "Def+"=400.0, "Def-"=400.0, "Offset"=0.0, "Slope"=218.45, "Type"=64, "Description"="Quadrupole 2 RF", "SettleT"=5.0}, {"Name"="Q2 DC", "Ch#"=5, "Min"=0.0, "Max"=1500.0, "Def+"=600.0, "Def-"=600.0, "Offset"=0.0, "Slope"=218.45, "Type"=64, "Description"="Quadrupole 2 DC", "SettleT"=5.0}, {"Name"="Q2 RR", "Ch#"=9, "Min"=0.0, "Max"=64000.0, "Def+"=32000.0, "Def-"=32000.0, "Offset"=32768.0, "Slope"=-1.0, "Type"=64, "Description"="Quadrupole 2 PW", "SettleT"=5.0}, {"Name"="M1 RF", "Ch#"=3, "Min"=0.0, "Max"=500.0, "Def+"=400.0, "Def-"=400.0, "Offset"=0.0, "Slope"=14.7, "Type"=6, "Description"="Multipole 1 RF", "SettleT"=5.0}, {"Name"="EV", "Ch#"=20, "Min"=-400.0, "Max"=400.0, "Def+"=0.0, "Def-"=0.0, "Offset"=32768.0, "Slope"=-65.7, "Type"=7, "Description"="Entrance voltage", "SettleT"=5.0}, {"Name"="ED", "Ch#"=21, "Min"=-400.0, "Max"=400.0, "Def+"=0.0, "Def-"=0.0, "Offset"=32768.0, "Slope"=-131.0, "Type"=7, "Description"="Not Used 1", "SettleT"=5.0}, {"Name"="M1", "Ch#"=19, "Min"=-400.0, "Max"=400.0, "Def+"=0.0, "Def-"=0.0, "Offset"=32768.0, "Slope"=-65.6, "Type"=7, "Description"="Multipole 1", "SettleT"=5.0}, {"Name"="L1", "Ch#"=18, "Min"=-400.0, "Max"=400.0, "Def+"=0.0, "Def-"=0.0, "Offset"=32760.0, "Slope"=-65.9, "Type"=7, "Description"="Multipole Len 1", "SettleT"=5.0}, {"Name"="M2", "Ch#"=22, "Min"=-400.0, "Max"=400.0, "Def+"=0.0, "Def-"=0.0, "Offset"=32768.0, "Slope"=-66.0, "Type"=7, "Description"="Multipole 2", "SettleT"=5.0}, {"Name"="L2", "Ch#"=11, "Min"=-400.0, "Max"=400.0, "Def+"=0.0, "Def-"=0.0, "Offset"=32768.0, "Slope"=-65.9, "Type"=7, "Description"="Multipole Len 2", "SettleT"=5.0}, {"Name"="PF", "Ch#"=12, "Min"=-400.0, "Max"=400.0, "Def+"=-16.0, "Def-"=16.0, "Offset"=32768.0, "Slope"=-65.8, "Type"=7, "Description"="Prefilter 1", "SettleT"=5.0}, {"Name"="Q1", "Ch#"=6, "Min"=-400.0, "Max"=400.0, "Def+"=-1.0, "Def-"=1.0, "Offset"=32755.0, "Slope"=-131.3, "Type"=11, "Description"="Quadrupole 1", "SettleT"=5.0}, {"Name"="CC L1", "Ch#"=13, "Min"=-400.0, "Max"=400.0, "Def+"=0.0, "Def-"=0.0, "Offset"=32768.0, "Slope"=-65.8, "Type"=7, "Description"="Collision Cell Lens 1", "SettleT"=5.0}, {"Name"="CC L2", "Ch#"=14, "Min"=-400.0, "Max"=400.0, "Def+"=-100.0, "Def-"=100.0, "Offset"=32768.0, "Slope"=-65.8, "Type"=7, "Description"="Collision Cell Lens 2", "SettleT"=5.0}, {"Name"="CC", "Ch#"=23, "Min"=-400.0, "Max"=400.0, "Def+"=-50.0, "Def-"=50.0, "Offset"=32768.0, "Slope"=-65.8, "Type"=7, "Description"="Collision Energy", "SettleT"=5.0}, {"Name"="CC AF", "Ch#"=10, "Min"=-400.0, "Max"=400.0, "Def+"=50.0, "Def-"=-50.0, "Offset"=32768.0, "Slope"=-65.8, "Type"=7, "Description"="Axial Field", "SettleT"=5.0}, {"Name"="CC L3", "Ch#"=15, "Min"=-400.0, "Max"=400.0, "Def+"=-52.5, "Def-"=52.5, "Offset"=32768.0, "Slope"=-65.7, "Type"=7, "Description"="Collision Cell Lens 3", "SettleT"=5.0}, {"Name"="CC L4", "Ch#"=16, "Min"=-400.0, "Max"=400.0, "Def+"=-72.5, "Def-"=72.5, "Offset"=32768.0, "Slope"=-65.7, "Type"=7, "Description"="Collision Cell Lens 4", "SettleT"=5.0}, {"Name"="Q2", "Ch#"=8, "Min"=-400.0, "Max"=400.0, "Def+"=-54.0, "Def-"=54.0, "Offset"=32756.0, "Slope"=-131.3, "Type"=11, "Description"="Quadrupole 2", "SettleT"=5.0}, {"Name"="ID", "Ch#"=17, "Min"=-400.0, "Max"=400.0, "Def+"=-400.0, "Def-"=400.0, "Offset"=32768.0, "Slope"=-65.8, "Type"=18, "Description"="Detector Deflector", "SettleT"=5.0}, {"Name"="DISC", "Ch#"=32, "Min"=10.0, "Max"=2000.0, "Def+"=20.0, "Def-"=20.0, "Offset"=-10.0, "Slope"=1.23, "Type"=18, "Description"="Discriminator", "SettleT"=5.0}, {"Name"="DV", "Ch#"=34, "Min"=0.0, "Max"=3500.0, "Def+"=500.0, "Def-"=500.0, "Offset"=0.0, "Slope"=0.615, "Type"=18, "Description"="Detector Voltage", "SettleT"=5.0}, {"Name"="DET horn", "Ch#"=200, "Min"=-5500.0, "Max"=5500.0, "Def+"=-1000.0, "Def-"=-1000.0, "Offset"=0.0, "Slope"=0.615, "Type"=16, "Description"="Detector Horn", "SettleT"=200.0}, {"Name"="LS400A", "Ch#"=36, "Min"=0.0, "Max"=420.0, "Def+"=420.0, "Def-"=420.0, "Offset"=0.0, "Slope"=8.4, "Type"=64, "Description"="Len Power Supply A +400", "SettleT"=5.0}, {"Name"="LS-400A", "Ch#"=37, "Min"=-420.0, "Max"=-55.0, "Def+"=-420.0, "Def-"=-420.0, "Offset"=-433.0, "Slope"=-8.4, "Type"=64, "Description"="Len Power Supply A -400", "SettleT"=5.0}, {"Name"="LS400B", "Ch#"=38, "Min"=0.0, "Max"=420.0, "Def+"=420.0, "Def-"=420.0, "Offset"=0.0, "Slope"=8.4, "Type"=64, "Description"="Len Power Supply B +400", "SettleT"=5.0}, {"Name"="LS-400B", "Ch#"=39, "Min"=-420.0, "Max"=-55.0, "Def+"=-420.0, "Def-"=-420.0, "Offset"=-433.0, "Slope"=-8.4, "Type"=64, "Description"="Len Power Supply B  -400", "SettleT"=5.0}, {"Name"="QPS800", "Ch#"=40, "Min"=110.0, "Max"=600.0, "Def+"=600.0, "Def-"=-600.0, "Offset"=0.0, "Slope"=4.25, "Type"=64, "Description"="Quad Power Supply +800", "SettleT"=5.0}, {"Name"="QPS-800", "Ch#"=41, "Min"=-600.0, "Max"=-110.0, "Def+"=600.0, "Def-"=-600.0, "Offset"=-433.0, "Slope"=-4.2, "Type"=64, "Description"="Quad Power Supply -800", "SettleT"=5.0}, {"Name"="DG", "Ch#"=26, "Min"=0.0, "Max"=5.0, "Def+"=0.4, "Def-"=0.4, "Offset"=0.0, "Slope"=3276.5, "Type"=32, "Description"="Drying Gas", "SettleT"=1000.0}, {"Name"="NG1", "Ch#"=27, "Min"=0.0, "Max"=5.0, "Def+"=0.0, "Def-"=0.0, "Offset"=0.0, "Slope"=3276.5, "Type"=32, "Description"="Nebulizer Gas 1", "SettleT"=1000.0}, {"Name"="HG1", "Ch#"=29, "Min"=0.0, "Max"=3.5, "Def+"=0.0, "Def-"=0.0, "Offset"=0.0, "Slope"=3276.5, "Type"=32, "Description"="Heating Gas 1", "SettleT"=1000.0}, {"Name"="NG2", "Ch#"=28, "Min"=0.0, "Max"=5.0, "Def+"=0.0, "Def-"=0.0, "Offset"=0.0, "Slope"=3276.5, "Type"=32, "Description"="Nebulizer Gas 2", "SettleT"=1000.0}, {"Name"="HG2", "Ch#"=30, "Min"=0.0, "Max"=3.5, "Def+"=0.0, "Def-"=0.0, "Offset"=0.0, "Slope"=3276.5, "Type"=32, "Description"="Heating Gas 2", "SettleT"=1000.0}, {"Name"="CC P", "Ch#"=43, "Min"=0.0, "Max"=5.0, "Def+"=0.0, "Def-"=0.0, "Offset"=0.0, "Slope"=3276.5, "Type"=6, "Description"="Collision Pressure", "SettleT"=3000.0}, {"Name"="SX", "Ch#"=42, "Min"=0.0, "Max"=5.0, "Def+"=0.0, "Def-"=0.0, "Offset"=0.0, "Slope"=3276.5, "Type"=32, "Description"="Source Exhaust", "SettleT"=1000.0}, {"Name"="ISV2", "Ch#"=204, "Min"=-6000.0, "Max"=6000.0, "Def+"=0.0, "Def-"=0.0, "Offset"=0.0, "Slope"=0.04, "Type"=34, "Description"="Ion Spray HV2", "SettleT"=200.0}, {"Name"="ISV1", "Ch#"=203, "Min"=-6000.0, "Max"=6000.0, "Def+"=0.0, "Def-"=0.0, "Offset"=0.0, "Slope"=0.04, "Type"=34, "Description"="Ion Spray HV1", "SettleT"=200.0}, {"Name"="CD", "Ch#"=202, "Min"=-5.0, "Max"=5.0, "Def+"=0.0, "Def-"=0.0, "Offset"=0.0, "Slope"=51.0, "Type"=34, "Description"="Corona Discharge", "SettleT"=2000.0}, {"Name"="CAP", "Ch#"=201, "Min"=-1100.0, "Max"=1100.0, "Def+"=0.0, "Def-"=0.0, "Offset"=0.0, "Slope"=0.22, "Type"=32, "Description"="Curtain Cap", "SettleT"=200.0}, {"Name"="HSID T", "Ch#"=81, "Min"=0.0, "Max"=350.0, "Def+"=200.0, "Def-"=200.0, "Offset"=0.0, "Slope"=1.0, "Type"=32, "Description"="HSID Temperature", "SettleT"=3000.0}, {"Name"="P1 T", "Ch#"=86, "Min"=0.0, "Max"=500.0, "Def+"=0.0, "Def-"=0.0, "Offset"=0.0, "Slope"=1.0, "Type"=32, "Description"="Probe 1 Temp", "SettleT"=3000.0}, {"Name"="P2 T", "Ch#"=84, "Min"=0.0, "Max"=500.0, "Def+"=0.0, "Def-"=0.0, "Offset"=0.0, "Slope"=1.0, "Type"=32, "Description"="Probe 2 Temp", "SettleT"=3000.0}], "Instrument"=["Q:\\Lab Common\\Default Startup Files\\Config Table\\Pending\\Config-Default-101026.c3n", "Ion Sniffer 03", "Ionics 3Q", "0", "0", "0", "0", "172.16.0.2", "T", "0", "2864776525 47721382", "2864776525 47721382", "2864776499 66657892", "5", "1"]}
  out "Q2 Res Lo":dbl[][](array[numeric])=[[0.0, 32500.0], [45.0, 33050.0], [514.1, 36000.77464788732], [585.4, 36552.29226361032], [933.6, 38547.70773638968], [1223.8, 40148.896492931395], [1456.0, 41430.06819957849], [1500.0, 41672.83975467096]] format="%.2f"
  out "Q2 Res Med":dbl[][](array[numeric])=[[0.0, 32600.0], [59.06, 33100.0], [175.13, 34050.0], [609.3, 36901.76174496644], [616.46, 36943.80872483221], [906.67, 38648.06208053691], [1254.9, 40749.39656707161], [1487.0, 42150.0], [1500.0, 42300.0]] format="%.2f"
  out "Q1 Res Lo":dbl[][](array[numeric])=[[0.0, 33265.24137931035], [59.06, 33900.54299922501], [175.13, 34950.975], [609.3, 38001.81208053691], [616.46, 38045.06040268456], [906.67, 39798.0067114094], [1254.9, 41899.39655117602], [1487.09, 43401.38461538462], [1500.0, 43600.0]] format="%.2f"
  out "Q1 Res Med":dbl[][](array[numeric])=[[0.0, 33265.24137931035], [59.06, 33900.54299922501], [175.13, 34950.975], [609.3, 38001.81208053691], [616.46, 38045.06040268456], [906.67, 39798.0067114094], [1254.9, 41899.39655117602], [1487.09, 43401.38461538462], [1500.0, 43600.0]] format="%.2f"
  out "Q2 Res Hi":dbl[][](array[numeric])=[[0.0, 32600.0], [59.06, 33100.0], [175.13, 34050.0], [609.3, 36901.76174496644], [616.46, 36943.80872483221], [906.67, 38648.06208053691], [1254.9, 40749.39656707161], [1487.0, 42150.0], [1500.0, 42300.0]] format="%.2f"
  out "Q2 Cal":dbl[][](array[numeric])=[[0.0, 0.0], [59.06, 8023.934304097528], [175.13, 24094.827090057508], [609.3, 84237.75059685535], [616.46, 85258.85953842459], [906.67, 125438.18017005036], [1254.9, 173704.72880677812], [1487.0, 205896.72157687077], [1500.0, 207852.79226600614]] format="%.2f"
  out "Q1 Res Hi":dbl[][](array[numeric])=[[0.0, 33265.24137931035], [59.06, 33900.54299922501], [175.13, 34950.975], [609.3, 38001.81208053691], [616.46, 38045.06040268456], [906.67, 39798.0067114094], [1254.9, 41899.39655117602], [1487.09, 43401.38461538462], [1500.0, 43600.0]] format="%.2f"
  out "Q1 Cal":dbl[][](array[numeric])=[[0.0, 0.0], [59.06, 8007.972231628852], [175.13, 24051.118700948115], [609.3, 84085.25564675158], [616.46, 85075.93195639057], [906.67, 125230.14589777726], [1254.9, 173425.601618889], [1487.09, 205562.74183429], [1500.0, 207349.59949474406]] format="%.2f"
  out "Max Mass":dbl=1600.0
  # "Instrument:\n0, File Name\n1, Serial #\n2, Model (contain LB for Leybold)\n3, Polarity Switching Time (mS)\n4, Source Switching Time (mS)\n5, CAD Gas Fill Time (mS)\n6, CAD Gas Evac Time (mS)\n7, IP Address\n8, Use DT Correction (T/F)\n9, Dead Time (nS)\n10, Q1 Oscillator Settings\n11, Q2 Oscillator Settings\n12, MP1 Oscillator Settings\n13, Pole Orientation\n14, Restore From Power Failure \n\nParameter Type:\n1, MR level\n2, Expt Level\n4, Compound Tab\n8, Resolution Tab\n16, DetectorTab\n32, Source Tab\n64, Reserved\n128, Reserved"
  # "Startup Mode:\n0, Startup\n1, Conventional Shutdown\n2. Total Shutdown"
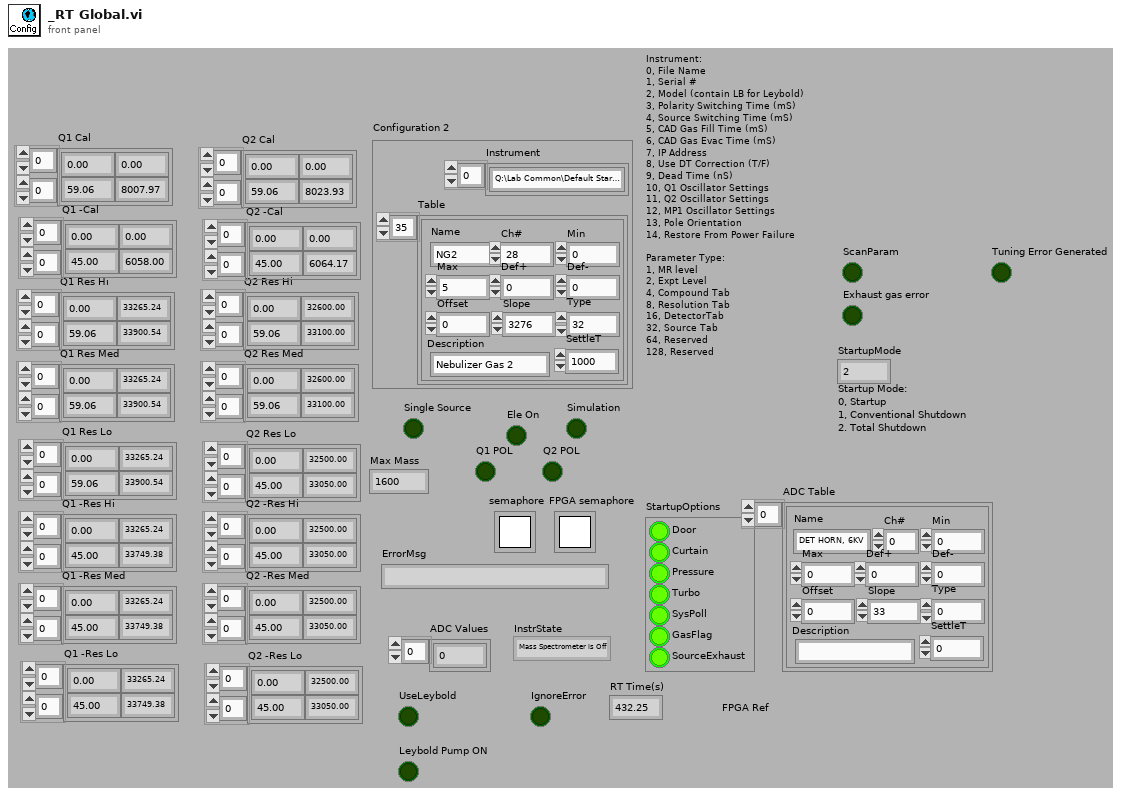
[diagram p1: front panel]
types:
  T1 = typedef "FPGA Typedef.ctl" = refnum<k20>
  T2 = typedef "Semaphore RefNum" = refnum<k1>
  T3 = typedef "_RT Instrument State.ctl" = enum16{"Initializing", "Mass Spectrometer is Off", "Starting Up", "Turning Power Off", "Going to Standby", "Roughing Pump Ready", "Turning Turbo Off", "Turbo Startup", "Turbopump Ready", "Checking Vacuum", "Going to Ready", "Ready", "Running", "Source Standby", "Lost Communication", "Shutting Down", "Fault", "24V Standby", "Go to 24V Standby", "Turbopump Ready-Waiting"}
  T4 = typedef "_RT Configuration 2.ctl" = cluster{"Name":string, "Ch#":u8, "Min":dbl, "Max":dbl, "Def+":dbl, "Def-":dbl, "Offset":dbl, "Slope":dbl, "Type":u8, "Description":string, "SettleT":dbl}
  T5 = typedef "_RT Startup Options.ctl" = cluster{"Door":bool, "Curtain":bool, "Pressure":bool, "Turbo":bool, "SysPoll":bool, "GasFlag":bool, "SourceExhaust":bool}
  T6 = typedef "_RT Instrument 2.ctl" = cluster{"Table":T4[], "Instrument":string[]}
diagram:
